vi "Action.vi"(8 "b":dbl, 10 "a":dbl, 11 "add in":refnum<class "multiple.lvclass">) -> (1 "result":dbl, 3 "add out":refnum<class "multiple.lvclass">)   [LabVIEW 2020, in "multiple.lvlib" / "multiple.lvclass"]
uses:
  multiple.lvclass
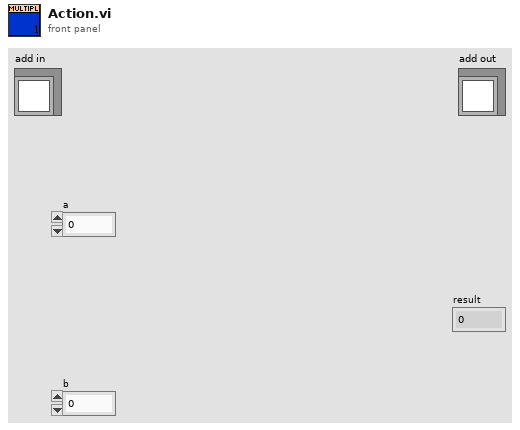
[diagram p1: front panel]
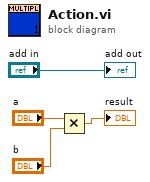
[diagram p0: block diagram]
diagram:
  n1 = Multiply(x="a", y="b") -> (x*y=→"result":dbl)
  "add out" <- "add in"
